vi "SysTest-Noise Generator.vi"() -> ()   [LabVIEW 2020]
uses:
  Signal Synthesis VIs/3rd Generation/XControls/Filter (G3)/Filter (G3).xctl
  Signal Synthesis VIs/3rd Generation/XControls/Level (G3)/Level Data.ctl
  Signal Synthesis VIs/3rd Generation/XControls/Level (G3)/Level Units (G3).ctl
  <vilib>/DAQmx/write.llb/DAQmx Write (Analog 1D DBL 1Chan NSamp).vi
  <vilib>/DAQmx/create/channels.llb/DAQmx Create Channel (AO-Voltage-Basic).vi
  <vilib>/DAQmx/configure/timing.llb/DAQmx Timing (Sample Clock).vi
  <vilib>/DAQmx/miscellaneous.llb/DAQmx Fill In Error Info.vi
  Signal Synthesis VIs/3rd Generation/XControls/Level (G3)/Level (G3).xctl
panel:
  in  "Frame size (s)":dbl=0.25
  out "Graph":dbl[](graph)
  in  "Stop":bool
  in  "Filter (G3)":T3(xcontrol)
  in  "Fs (Hz)":dbl=100000.0
  in  "Level (dB re 1V)":dbl=-20.0
  in  "Channel":tag
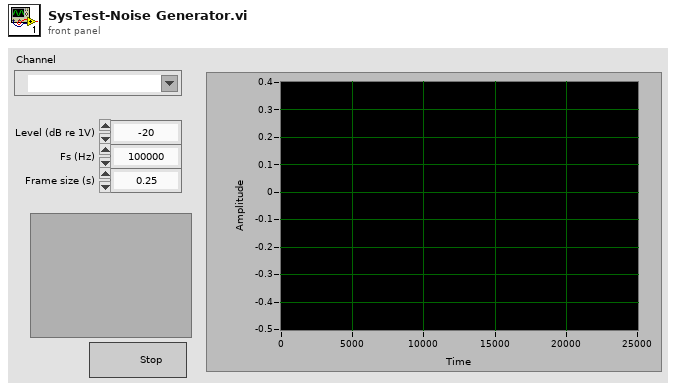
[diagram p1: front panel]
types:
  T1 = typedef "Filter (G3).xctl/Filter Type.ctl" = enum16{"OFF", "Lowpass", "Highpass", "Bandpass", "Bandstop"}
  T2 = typedef "Filter-Bandwidth Units.ctl" = enum16{"Linear", "Octaves", "Min-Max"}
  T3 = cluster{"Type":T1, "CF (kHz)":dbl, "BW (kHz)":dbl, "Cascade":bool, "Quadrature":bool, "Scale Factor":dbl, "Stages":cluster{"IIR Filter":cluster{"filter structure":enum32{"IIR 2nd Order", "IIR 4th Order"}, "Reverse Coefficients":dbl[], "Forward Coefficients":dbl[]}, "State":dbl[]}[], "Class":enum16{"Elliptic", "Butterworth"}, "Order":i32, "BWUnits":T2}
  T4 = typedef "Level (G3).xctl/Level Units (G3).ctl" = enum16{"dB atten", "dB SPL", "dB re 1 Vrms", "dB V/Hz½", "mW", "dB HL", "Volts", "dB mW"}
  T5 = typedef "Level (G3).xctl/Level Data.ctl" = cluster{"Level":dbl, "Units":T4, "Max":dbl, "Data":cluster{"Multiplier":dbl, "Cal File":path, "Cal":cluster{"Freq (Hz)":dbl[], "Mag (dB SPL)":dbl[], "Phase (deg)":dbl[]}, "audiogram":path}}
  T6 = typedef "Noise (G3).ctl" = cluster{"Properties":T7, "Data":T8}
  T7 = typedef "Noise (G3).Properties.ctl" = cluster{"InvFilt":bool, "Aweight":bool, "Seed":i32, "Tokens":i32, "Brickwall":bool}
  T8 = typedef "Noise (G3).Data.ctl" = cluster{"TokenNum":i32}
  T9 = typedef "Filter (G3).xctl/Filter Data.ctl" = cluster{"Type":T1, "CF (kHz)":dbl, "BW (kHz)":dbl, "Cascade":bool, "Quadrature":bool, "Scale Factor":dbl, "Stages":cluster{"IIR Filter":cluster{"filter structure":enum32{"IIR 2nd Order", "IIR 4th Order"}, "Reverse Coefficients":dbl[], "Forward Coefficients":dbl[]}, "State":dbl[]}[], "Class":enum16{"Elliptic", "Butterworth"}, "Order":i32, "BWUnits":T2}
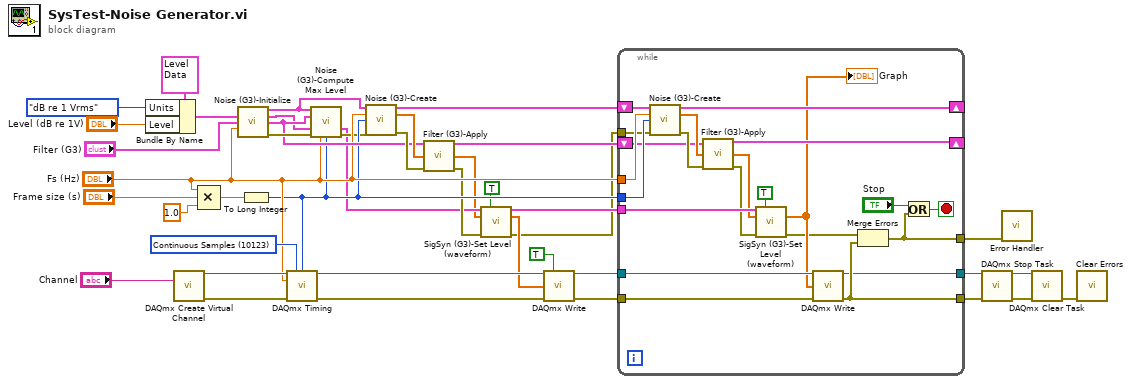
[diagram p0: block diagram]
diagram:
  w37 = 10123 items=["Finite Samples"=10178, "Continuous Samples"=10123, "Hardware Timed Single Point"=12522] ("sample mode")
  n1 = Bundle By Name(cluster=T5 {"Level"=0.0, "Units"=enum."dB atten", "Max"=0.0, "Data"={"Multiplier"=0.0, "Cal File"=path "", "Cal"={"Freq (Hz)"=[], "Mag (dB SPL)"=[], "Phase (deg)"=[]}, "audiogram"=path ""}} ("Level"), "Units"=Level_Units_(G3)."dB re 1 Vrms", "Level"="Level (dB re 1V)") -> (w30:T5)
  n2 = call-poly <vilib>:"DAQmx Create Virtual Channel.vi"("physical channels"="Channel") -> ("task out"=w38:refnum<k21>, "error out"=w39:errorcluster)  [unwired: 13 in]
  n3 = Compound Arithmetic op=MULTIPLY("Fs (Hz)", "Frame size (s)", 1.0 ("value")) -> (w36:dbl)
  n4 = call "Noise (G3)-Initialize.vi"("Level"=w30, "Filter"="Filter (G3)", "Sampling rate (Hz)"="Fs (Hz)") -> ("Noise Out"=w9:T6, "Level Out"=w12:T5, "Filter Out"=w13:T9, "error out"=w14:errorcluster)  [unwired: 8 in, 1 out]
  n5 = To Long Integer(number=w36) -> (32bit integer=w10:i32)
  n6 = call-poly <vilib>:"DAQmx Timing.vi"("task/channels in"=w38, "sample mode"=w37, "samples per channel"=w10, "rate"="Fs (Hz)", "error in"=w39) -> ("task out"=w34:refnum<k21>, "error out"=w35:errorcluster)  [unwired: 9 in]
  n7 = call "Noise (G3)-Compute Max Level.vi"("Noise Params"=w9, "Filter"=w13, "Level"=w12, "error in (no error)"=w14, "Sampling Rate (Hz)"="Fs (Hz)", "Npts"=w10) -> ("Level out"=w6:T5, "error out"=w8:errorcluster)  [unwired: 7 in, 1 out]
  n8 = call "Noise (G3)-Create.vi"("Noise In"=w9, "Sampling Rate (Hz)"="Fs (Hz)", "Npts"=w10, "error in (no error)"=w8) -> ("Noise Out"=w25:T6, "Waveform"=w16:dbl[], "error out"=w17:errorcluster)  [unwired: 9 in]
  n9 = call "Filter (G3)-Apply.vi"("Filter"=w13, "X"=w16, "error in (no error)"=w17) -> ("Filter out"=w15:T9, "Filtered X"=w3:dbl[], "error out"=w7:errorcluster)  [unwired: 10 in]
  n10 = call "SigSyn (G3)-Set Level (waveform).vi"("Level"=w6, "Apply multiplier? (F)"=TRUE, "Waveform in"=w3, "error in (no error)"=w7) -> ("Level out"=w5:T5, "Waveform out"=w4:dbl[], "error out"=w1:errorcluster)  [unwired: 7 in, 2 out]
  n11 = call-poly <vilib>:"DAQmx Write.vi"("task/channels in"=w34, "auto start"=TRUE, "data"=w4, "error in"=w35) -> ("task out"=w26:refnum<k21>, "error out"=w27:errorcluster)  [unwired: 9 in, 1 out]
  n12 = while {
    tunnel: w27 -> [w63]
    tunnel: w26 -> [w62]
    shift-right: [w60] -> _
    shift-left: w25 -> [w61]
    tunnel: "Fs (Hz)" -> [w59]
    tunnel: w10 -> [w58]
    tunnel: w1 -> [w57]
    tunnel: [w56] -> w23
    tunnel: [w53] -> w22
    tunnel: [w52] -> w21
    shift-right: [w48] -> _
    shift-left: w15 -> [w49]
    tunnel: w5 -> [w47]
    stop <- w54 stop-if-true
    n13 = call "Noise (G3)-Create.vi"("Noise In"=w61, "Sampling Rate (Hz)"=w59, "Npts"=w58, "error in (no error)"=w57) -> ("Noise Out"=w60:T6, "Waveform"=w50:dbl[], "error out"=w51:errorcluster)  [unwired: 9 in]
    n14 = call "Filter (G3)-Apply.vi"("Filter"=w49, "X"=w50, "error in (no error)"=w51) -> ("Filter out"=w48:T9, "Filtered X"=w46:dbl[], "error out"=w43:errorcluster)  [unwired: 10 in]
    n15 = call "SigSyn (G3)-Set Level (waveform).vi"("Level"=w47, "Apply multiplier? (F)"=TRUE, "Waveform in"=w46, "error in (no error)"=w43) -> ("Waveform out"=w45:dbl[], "error out"=w42:errorcluster)  [unwired: 7 in, 3 out]
    "Graph" <- w45
    n16 = call-poly <vilib>:"DAQmx Write.vi"("task/channels in"=w62, "data"=w45, "error in"=w63) -> ("task out"=w52:refnum<k21>, "error out"=w53:errorcluster)  [unwired: 10 in, 1 out]
    n17 = Merge Errors(w42, w53) -> (w56:errorcluster)
    n18 = Or(x="Stop", y=w56) -> (x .or. y?=w54:bool)
  }
  n19 = call <vilib>:"DAQmx Stop Task.vi"("task/channels in"=w21, "error in"=w22) -> ("task out"=w20:refnum<k21>, "error out"=w19:errorcluster)  [unwired: 12 in]
  n20 = call "Error Handler.vi"("error in (no error)"=w23) -> ()  [unwired: 13 in, 2 out]
  n21 = call <vilib>:"DAQmx Clear Task.vi"("task in"=w20, "error in"=w19) -> ("error out"=w18:errorcluster)  [unwired: 13 in]
  n22 = call <vilib>:"Clear Errors.vi"("error in (no error)"=w18) -> ()  [unwired: 5 in, 2 out]
